vi "PI Controller.vi"(1 "Control Signal Range":cluster{"u_max":dbl, "u_min":dbl}, 2 "PI Parameters":cluster{"Kp":dbl, "Ti [s]":dbl}, 3 "Process":T1, 4 "Ts [s]":dbl) -> (0 "Output":dbl)   [LabVIEW 2022 SP3]
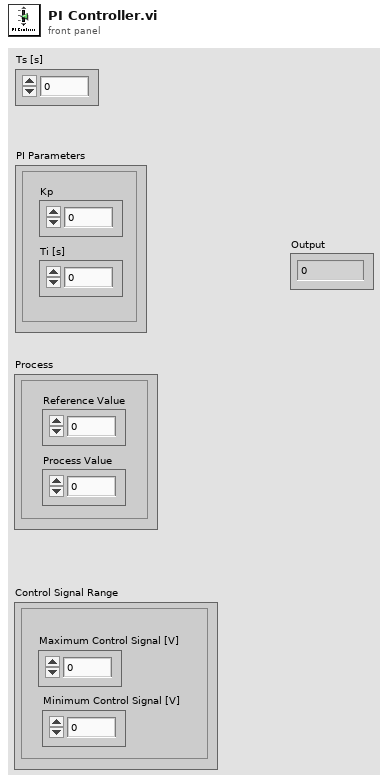
[diagram p1: front panel]
types:
  T1 = cluster{"Reference Value":dbl, "Process Value":dbl}
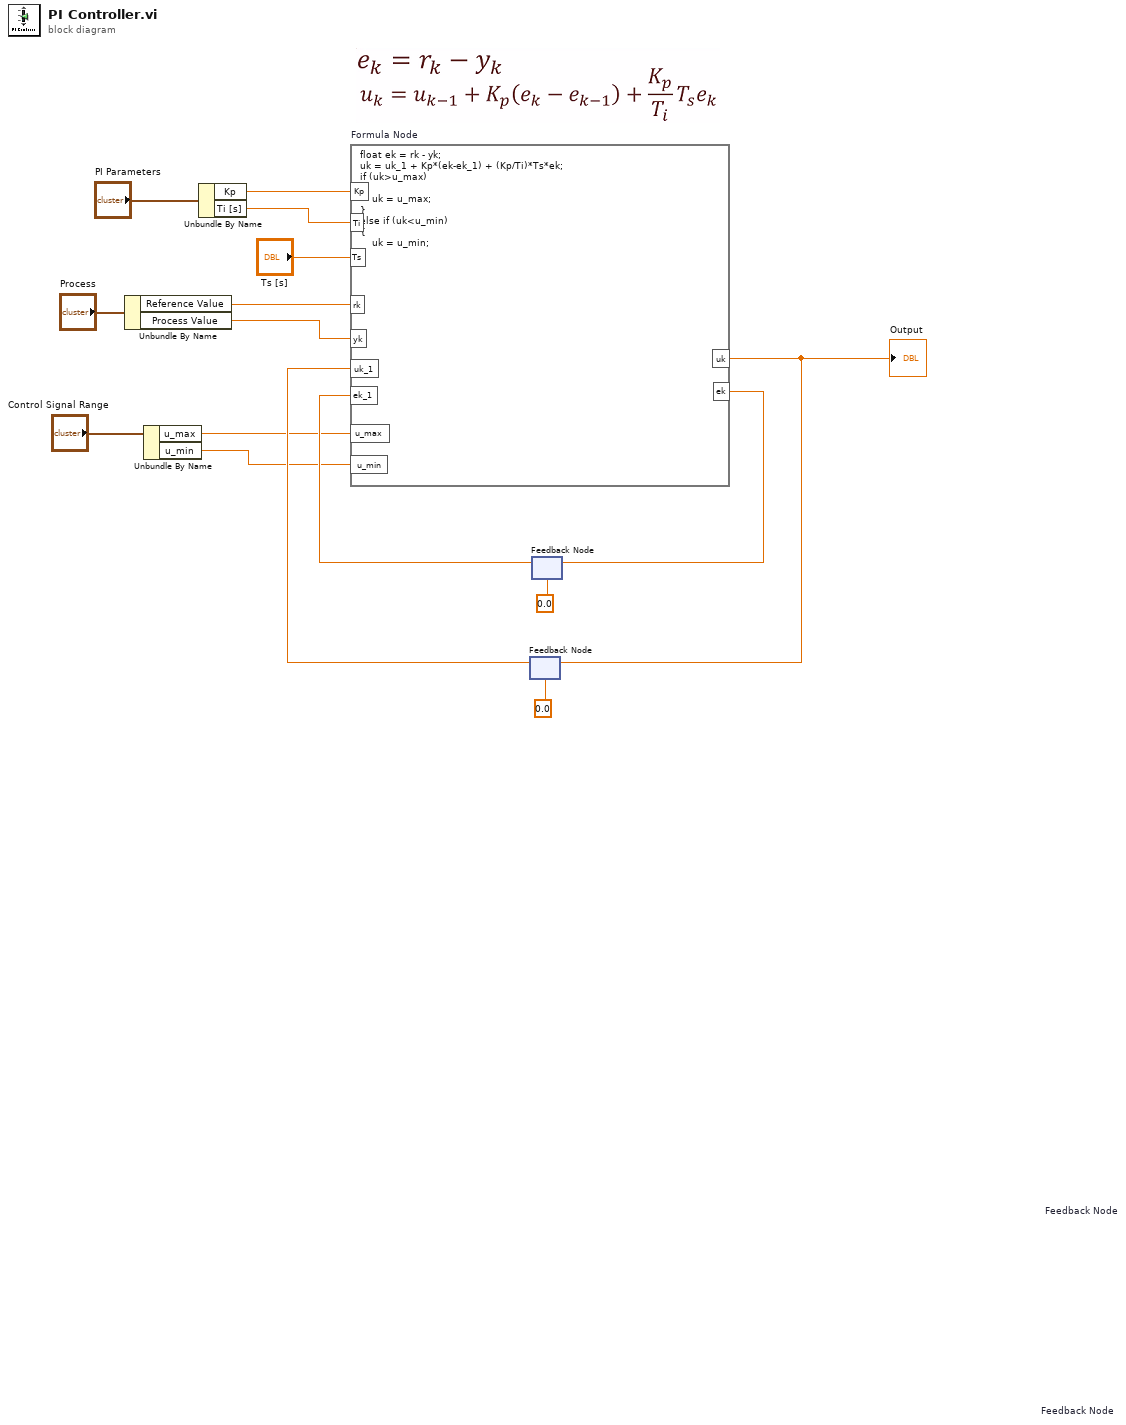
[diagram p0: block diagram]
diagram:
  n1 = Unbundle By Name "Unbundle By Name"("Process") -> ("Reference Value"=w5:dbl, "Process Value"=w4:dbl)
  n2 = Unbundle By Name "Unbundle By Name"("Control Signal Range") -> ("u_max"=w2:dbl, "u_min"=w1:dbl)
  n3 = Unbundle By Name "Unbundle By Name"("PI Parameters") -> ("Kp"=w15:dbl, "Ti [s]"=w14:dbl)
  n4 = feedback #1 "Feedback Node"(0.0 ("uk")) -> (w9:dbl)
  n5 = feedback #2 "Feedback Node"(0.0) -> (w11:dbl)
  n6 = formula code="float ek = rk - yk;\nuk = uk_1 + Kp*(ek-ek_1) + (Kp/Ti)*Ts*ek;\nif (uk>u_max)\n{\n    uk = u_max;\n}\nelse if (uk<u_min)\n{\n    uk = u_min;\n}"("rk"=w5, "yk"=w4, "uk_1"=w9, "Ti"=w14, "Kp"=w15, "Ts"="Ts [s]", "ek_1"=w11, "u_max"=w2, "u_min"=w1) -> ("uk"=w10:dbl, "ek"=w12:dbl)
  "Output" <- w10
  n7 = feedback-in #1(w10) -> ()
  n8 = feedback-in #2(w12) -> ()
